vi "CalcBouncerGate.vi"(9 "Bouncer Settings":T1, 10 "SampClk.Rate":dbl) -> (1 "Bouncer Waveform":waveform(dbl), 2 "High time":dbl, 3 "low time":dbl)   [LabVIEW 2011]
uses:
  BouncerParameters.ctl
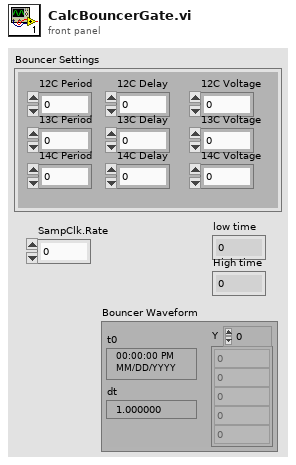
[diagram p1: front panel]
types:
  T1 = typedef "BouncerParameters.ctl" = cluster{"12C Period":dbl, "12C Delay":dbl, "12C Voltage":dbl, "13C Period":dbl, "13C Delay":dbl, "13C Voltage":dbl, "14C Period":dbl, "14C Delay":dbl, "14C Voltage":dbl}
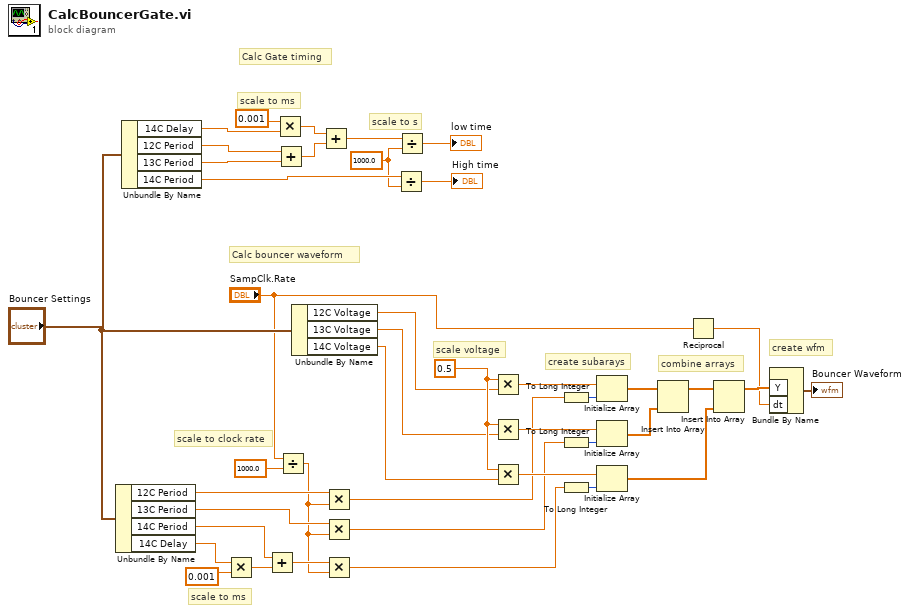
[diagram p0: block diagram]
diagram:
  w12 = 1000.0 ("y")
  w38 = 0.5 ("y")
  # "Calc bouncer waveform"
  # "Calc Gate timing"
  # "create wfm"
  # "combine arrays"
  # "create subarays"
  # "scale voltage"
  # "scale to clock rate"
  # "scale to ms"
  # "scale to s"
  # "scale to ms"
  n1 = Unbundle By Name("Bouncer Settings") -> ("12C Period"=w30:dbl, "13C Period"=w29:dbl, "14C Period"=w21:dbl, "14C Delay"=w18:dbl)
  n2 = Unbundle By Name("Bouncer Settings") -> ("14C Delay"=w10:dbl, "12C Period"=w15:dbl, "13C Period"=w16:dbl, "14C Period"=w17:dbl)
  n3 = Multiply(x=w18, y=0.001) -> (x*y=w19:dbl)
  n4 = Add(x=w21, y=w19) -> (x+y=w42:dbl)
  n5 = Multiply(x=0.001 ("y"), y=w10) -> (x*y=w14:dbl)
  n6 = Add(x=w15, y=w16) -> (x+y=w13:dbl)
  n7 = Divide(x="SampClk.Rate", y=1000.0) -> (x/y=w2:dbl)
  n8 = Unbundle By Name("Bouncer Settings") -> ("12C Voltage"=w28:dbl, "13C Voltage"=w27:dbl, "14C Voltage"=w26:dbl)
  n9 = Add(x=w14, y=w13) -> (x+y=w11:dbl)
  n10 = Multiply(x=w30, y=w2) -> (x*y=w34:dbl)
  n11 = Multiply(x=w29, y=w2) -> (x*y=w33:dbl)
  n12 = Multiply(x=w42, y=w2) -> (x*y=w32:dbl)
  n13 = Divide(x=w17, y=w12) -> (x/y=→"High time":dbl)
  n14 = Divide(x=w11, y=w12) -> (x/y=→"low time":dbl)
  n15 = Multiply(x=w38, y=w28) -> (x*y=w40:dbl)
  n16 = Multiply(x=w38, y=w27) -> (x*y=w39:dbl)
  n17 = Multiply(x=w38, y=w26) -> (x*y=w41:dbl)
  n18 = To Long Integer(number=w34) -> (32bit integer=w23:i32)
  n19 = To Long Integer(number=w33) -> (32bit integer=w24:i32)
  n20 = To Long Integer(number=w32) -> (32bit integer=w25:i32)
  n21 = Initialize Array(w40, w23) -> (w5:dbl[])
  n22 = Initialize Array(w39, w24) -> (w37:dbl[])
  n23 = Initialize Array(w41, w25) -> (w36:dbl[])
  n24 = Insert Into Array(array=w5, new element=w37) -> (w4:dbl[])  [unwired: 1 in]
  n25 = Reciprocal(x="SampClk.Rate") -> (1/x=w31:dbl)
  n26 = Insert Into Array(array=w4, new element=w36) -> (w35:dbl[])  [unwired: 1 in]
  n27 = Bundle By Name("Y"=w35, "dt"=w31) -> (→"Bouncer Waveform":waveform(dbl))  [unwired: 1 out]
